vi "Get Angle and Magnitude.vi"(8 "YGoal":sgl, 9 "XGoal":sgl, 10 "Y":sgl, 11 "X":sgl) -> (0 "delta Y":sgl, 1 "delta X":sgl, 2 "Magnitude":sgl, 3 "Angle Out (rad)":sgl)   [LabVIEW 2016]
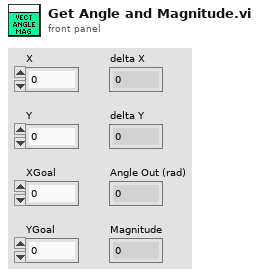
[diagram p1: front panel]
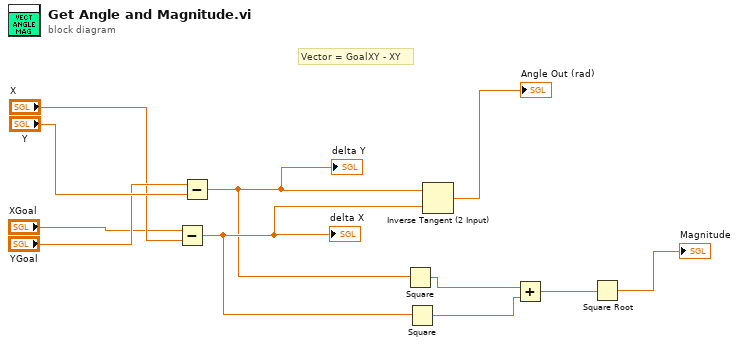
[diagram p0: block diagram]
diagram:
  # "Vector = GoalXY - XY"
  n1 = Subtract(x="XGoal", y="X") -> (x-y=w7:sgl)
  "delta X" <- w7
  n2 = Subtract(x="YGoal", y="Y") -> (x-y=w6:sgl)
  "delta Y" <- w6
  n3 = Square(x=w6) -> (x^2=w8:sgl)
  n4 = Square(x=w7) -> (x^2=w9:sgl)
  n5 = Inverse Tangent (2 Input)(1:w7, 2:w6) -> (0:→"Angle Out (rad)":sgl)
  n6 = Add(x=w8, y=w9) -> (x+y=w10:sgl)
  n7 = Square Root(x=w10) -> (sqrt(x)=→"Magnitude":sgl)
